vi "FalconVelocityToRPM.vi"(4 "raw sensor units / 100 ms":dbl) -> (1 "RPM":dbl)   [LabVIEW 2019]
panel:
  in  "constant":dbl=0.2478966 format="%#_13g"
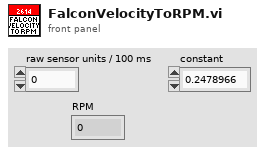
[diagram p1: front panel]
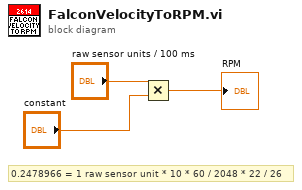
[diagram p0: block diagram]
diagram:
  # "0.2478966 = 1 raw sensor unit * 10 * 60 / 2048 * 22 / 26"
  n1 = Multiply(x="raw sensor units / 100 ms", y="constant") -> (x*y=→"RPM":dbl)
